vi "encoder rotation.vi"(9 "Reset Encoder":bool, 10 "Switch value":bool, 11 "Voltage":dbl) -> (2 "Offset":dbl format="%#_13g", 3 "Angle(rad)":dbl, 5 "Count":dbl)   [LabVIEW 2015]
uses:
  <vilib>/ptbypt/NI_PtbyPt.lvlib
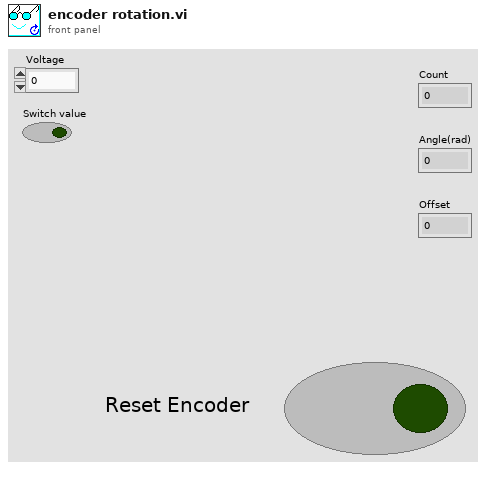
[diagram p1: front panel]
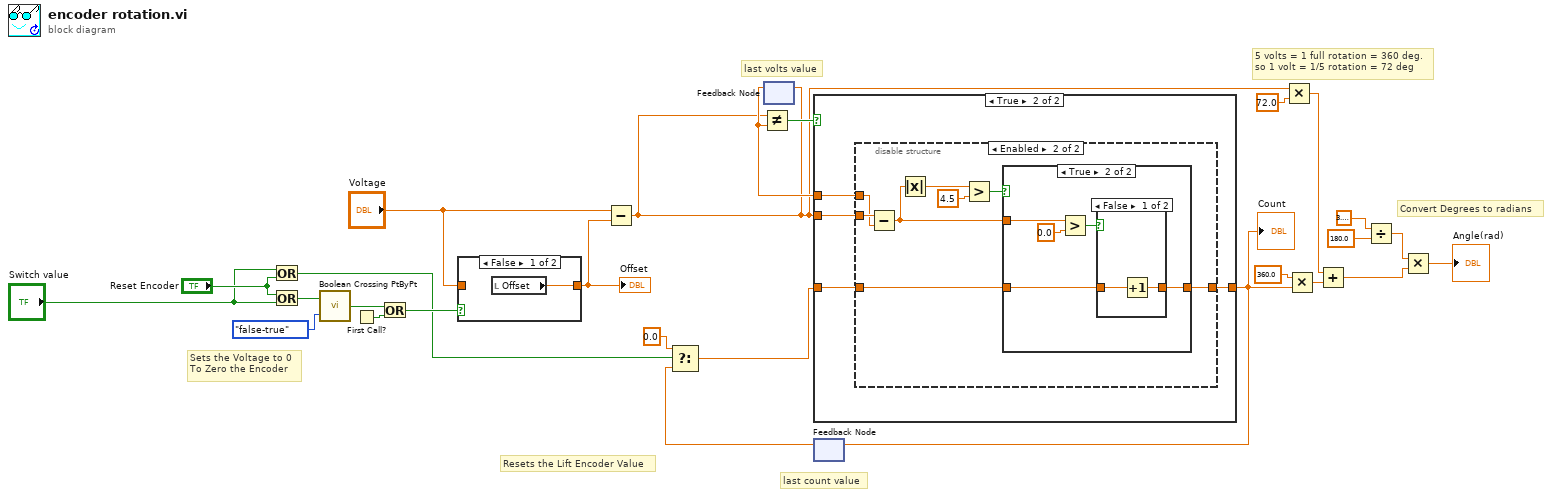
[diagram p0: block diagram]
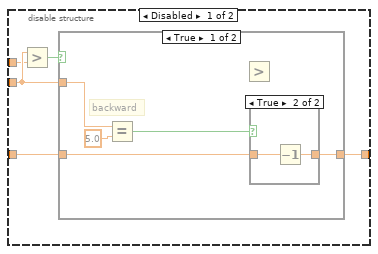
[diagram p4: hidden frame]
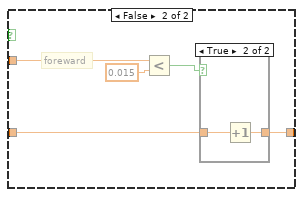
[diagram p6: hidden frame]
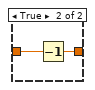
[diagram p9: hidden frame]
diagram:
  # "Resets the Lift Encoder Value"
  # "Sets the Voltage to 0 \nTo Zero the Encoder"
  # "5 volts = 1 full rotation = 360 deg.\nso 1 volt = 1/5 rotation = 72 deg"
  # "Convert Degrees to radians"
  # "last volts value"
  # "last count value"
  n1 = Or(x="Switch value", y="Reset Encoder") -> (x .or. y?=w3:bool)
  n2 = Or(x="Reset Encoder", y="Switch value") -> (x .or. y?=w10:bool)
  n3 = call <vilib>:"Boolean Crossing PtByPt.vi"("direction"=enum16{"either", "false-true", "true-false"}."false-true", "input"=w10) -> ("crossing"=w5:bool)  [unwired: 1 in]
  n4 = First Call?() -> (First Call?: T/F=w7:bool)
  n5 = Or(x=w5, y=w7) -> (x .or. y?=w8:bool)
  n6 = case shown="False" w8 {
    tunnel: [w27 w28] -> w4
    tunnel: "Voltage" -> [_ w28]
    frame False {
      n7 = local read "Offset"() -> (w27:dbl)
    }
    frame True {
    }
  }
  "Offset" <- w4
  n8 = Subtract(x="Voltage", y=w4) -> (x-y=w11:dbl)
  n9 = feedback #1() -> (w25:dbl)  [unwired: 1 in]
  n10 = Not Equal?(x=w11, y=w25) -> (x != y?=w26:bool)
  n11 = feedback-in #1(w11) -> ()
  n12 = feedback #2() -> (w13:dbl)  [unwired: 1 in]
  n13 = Select(t=0.0, s=w3, f=w13) -> (s? t:f=w12:dbl)
  n14 = case shown="True" w26 {
    tunnel: w12 -> [w29 w31]
    tunnel: w11 -> [_ w32]
    tunnel: [w29 w33] -> w24
    tunnel: w25 -> [_ w30]
    frame False {
    }
    frame True {
      n15 = disable-structure shown="Enabled" {
        disable-tunnel: [w38 w56] -> w33
        disable-tunnel: w32 -> [w36 w63]
        disable-tunnel: w31 -> [w35 w57]
        disable-tunnel: w30 -> [w34 w62]
        frame Disabled {
          n16 = Greater?(x=w36, y=w34) -> (0:w37:bool)
          n17 = case shown="True" w37 {
            tunnel: w36 -> [w42 w51]
            tunnel: w35 -> [w44 w50]
            tunnel: [w43 w49] -> w38
            frame True {
              # "backward"
              n18 = Equal?(x=w42, y=5.0) -> (x = y?=w40:bool)
              n19 = Greater?() -> (y=w39:dbl)  [unwired: 1 in, 1 out]
              n20 = case shown="True" w40 {
                tunnel: [w45 w47] -> w43
                tunnel: w44 -> [w45 w46]
                frame False {
                }
                frame True {
                  n21 = Decrement(x=w46) -> (x-1=w47:dbl)
                }
              }
            }
            frame False {
              # "foreward"
              n22 = Less?(x=w51, y=0.015) -> (x < y?=w48:bool)
              n23 = case shown="True" w48 {
                tunnel: [w53 w55] -> w49
                tunnel: w50 -> [w53 w54]
                frame False {
                }
                frame True {
                  n24 = Increment(x=w54) -> (x+1=w55:dbl)
                }
              }
            }
          }
        }
        frame Enabled {
          n25 = Subtract(x=w63, y=w62) -> (x-y=w58:dbl)
          n26 = Absolute Value(x=w58) -> (abs(x)=w61:dbl)
          n27 = Greater?(x=w61, y=4.5) -> (0:w59:bool)
          n28 = case shown="True" w59 {
            tunnel: w58 -> [_ w68]
            tunnel: w57 -> [w64 w66]
            tunnel: [w64 w65] -> w56
            frame False {
            }
            frame True {
              n29 = Greater?(x=w68, y=0.0) -> (0:w67:bool)
              n30 = case shown="False" w67 {
                tunnel: w66 -> [w71 w73]
                tunnel: [w70 w72] -> w65
                frame False {
                  n31 = Increment(x=w71) -> (x+1=w70:dbl)
                }
                frame True {
                  n32 = Decrement(x=w73) -> (x-1=w72:dbl)
                }
              }
            }
          }
        }
      }
    }
  }
  "Count" <- w24
  n33 = feedback-in #2(w24) -> ()
  n34 = Multiply(x=w11, y=72.0) -> (x*y=w21:dbl)
  n35 = Multiply(x=360.0, y=w24) -> (x*y=w20:dbl)
  n36 = Add(x=w21, y=w20) -> (x+y=w19:dbl)
  n37 = Divide(x=3.141592653589793, y=180.0) -> (x/y=w16:dbl)
  n38 = Multiply(x=w16, y=w19) -> (x*y=→"Angle(rad)":dbl)
